vi "magspec simple reader BELLA.vi"(9 "Image Name":string, 10 "magspec letter":string, 11 "File Path":path) -> (3 "Refnum out":T2)   [LabVIEW 2011]
uses:
  <vilib>/vision/Image Controls.llb/IMAQ Image.ctl
  <vilib>/vision/NI_Vision_Development_Module.lvlib
panel:
  out "Size & Order # 2":T1={"X Size"=3, "Y Size"=3, "Order #"=4}
  in  "Median Size (odd please)":i32=3
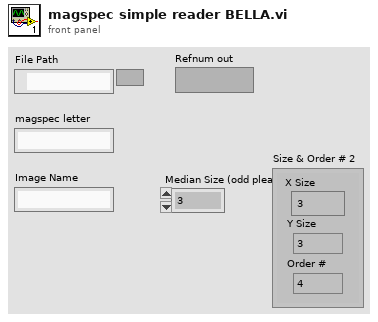
[diagram p1: front panel]
types:
  T1 = cluster{"X Size":i32, "Y Size":i32, "Order #":i32}
  T2 = typedef "IMAQ Image.ctl" = refnum<image>
  T3 = typedef "Image Type" = u32
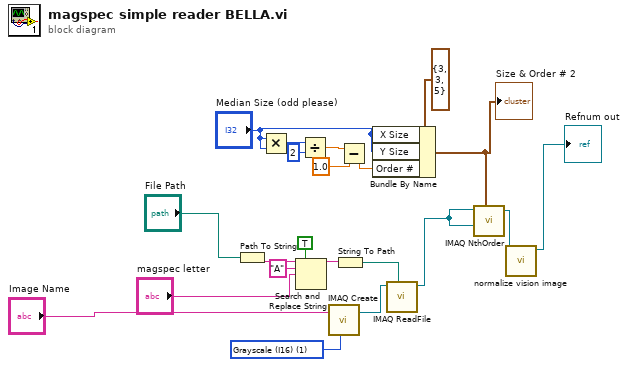
[diagram p0: block diagram]
diagram:
  w13 = T3 1 items=["Grayscale (U8)", "Grayscale (I16)", "Grayscale (SGL)", "Complex (CSG)", "RGB (U32)", "HSL (U32)", "RGB (U64)", "Grayscale (U16)"] ("Image Type")
  n1 = Path To String(path="File Path") -> (string=w15:string)
  n2 = Multiply(x="Median Size (odd please)", y="Median Size (odd please)") -> (x*y=w8:i32)
  n3 = Search and Replace String(replace all?=TRUE ("replace all? (F)"), input string=w15, search string="A", replace string="magspec letter") -> (result string=w18:string)  [unwired: 4 in, 3 out]
  n4 = Divide(x=w8, y=2) -> (x/y=w6:dbl)
  n5 = call "IMAQ Create"("Image Name"="Image Name", "Image Type"=w13) -> ("New Image"=w20:T2)  [unwired: 3 in, 1 out]
  n6 = String To Path(string=w18) -> (path=w19:path)
  n7 = Subtract(x=w6, y=1.0) -> (x-y=w2:dbl)
  n8 = Bundle By Name(cluster=T1 {"X Size"=3, "Y Size"=3, "Order #"=5} ("Size & Order #"), "X Size"="Median Size (odd please)", "Y Size"="Median Size (odd please)", "Order #"=w2) -> (w1:T1)
  "Size & Order # 2" <- w1
  n9 = call "IMAQ ReadFile"("File Path"=w19, "Image"=w20) -> ("Image Out"=w11:T2)  [unwired: 5 in, 4 out]
  n10 = call "IMAQ NthOrder"("Image Src"=w11, "Size & Order #"=w1, "Image Dst"=w11) -> ("Image Dst Out"=w10:T2)  [unwired: 4 in, 1 out]
  n11 = call "normalize vision image.vi"("Refnum in"=w10) -> ("Refnum out"=→"Refnum out":T2)  [unwired: 8 in, 2 out]
